vi "RSZVB Get Pressed Soft Key.vi"(8 "error in (no error)":errorcluster {"code" format="%.0x"}, 11 "VISA session":refnum<visa-resource-name>) -> (0 "error out":errorcluster {"code" format="%.0x"}, 1 "Label":string, 2 "Key Number":i32, 3 "dup VISA session":refnum<visa-resource-name>)   [LabVIEW 2011]
doc: "This VI returns the number and label of the softkey pressed most recently. If no softkey was pressed, the string 0,'' is returned.\n\nRemote-control command(s):\n:SYSTem:USER:FKEY?"
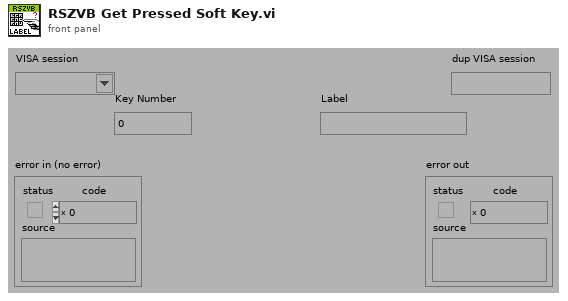
[diagram p1: front panel]
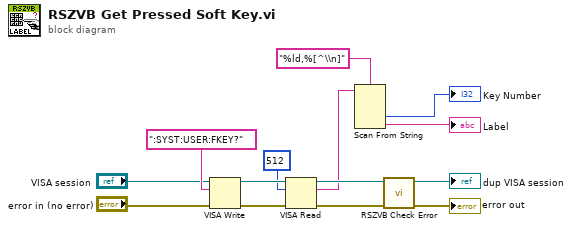
[diagram p0: block diagram]
diagram:
  n1 = VISA Write(VISA resource name="VISA session", write buffer=":SYST:USER:FKEY?", error in (no error)="error in (no error)") -> (VISA resource name out=w13:refnum<visa-resource-name>, error out=w12:errorcluster)  [unwired: 1 out]
  n2 = VISA Read(VISA resource name=w13, byte count=u32 512 ("byte count (0)"), error in (no error)=w12) -> (VISA resource name out=w11:refnum<visa-resource-name>, read buffer=w4:string, error out=w10:errorcluster)  [unwired: 1 out]
  n3 = Scan From String(format string="%ld,%[^\\n]", input string=w4) -> (output 1=→"Key Number":i32, output 2=→"Label":string)  [unwired: 4 in, 3 out]
  n4 = call "RSZVB Check Error.vi"("error in (no error)"=w10, "VISA session"=w11) -> ("error out"=→"error out":errorcluster, "dup VISA session"=→"dup VISA session":refnum<visa-resource-name>)  [unwired: 8 in]
